vi "D-O Status Module.vi"(8 "error in (no error)":errorcluster, 11 "?":T1={"State"=enum."Idle", "Start Time"=timestamp(0 s since 1904-01-01), "Configuration"={"D-O State"=0, "Cycle Period"=0.0, "DAQmx Task Name"="", "Input Channel Tag Name"=""}, "Current Time"=timestamp(0 s since 1904-01-01), "First Iteration"=FALSE, "Data"={"D-O State"=0}, "Process Name"="", "Pump On?"=enum."Off", "Output Error"=FALSE, "Log Started"=FALSE} {"Data"."D-O State" items=["Default", "On", "Off", "Not Initialized"]; "Configuration"."D-O State" items=["Default", "On", "Off", "Not Initialized"]}) -> (0 "error out":errorcluster, 3 "State out":T1={"State"=enum."Idle", "Start Time"=timestamp(0 s since 1904-01-01), "Configuration"={"D-O State"=0, "Cycle Period"=0.0, "DAQmx Task Name"="", "Input Channel Tag Name"=""}, "Current Time"=timestamp(0 s since 1904-01-01), "First Iteration"=FALSE, "Data"={"D-O State"=0}, "Process Name"="", "Pump On?"=enum."Off", "Output Error"=FALSE, "Log Started"=FALSE} {"Data"."D-O State" items=["Default", "On", "Off", "Not Initialized"]; "Configuration"."D-O State" items=["Default", "On", "Off", "Not Initialized"]})   [LabVIEW 2018, in "D-O Module.lvlib"]
uses:
  D-O Module.lvlib
  Ismatec ISM 831C/Ismatec ISM 831C.lvlib
  Masterflex 7550-30/Masterflex 7550-30.lvlib
  Tag VIs/Tag FGV Operation Enum.ctl
  Shared Variables/Dynamic Shared Variables.lvlib
  Measure Instrument/D-O Module Engine.lvlib
  Tacmina QI/Tacmina QI.lvlib
  KNF Pump/KNF SIMDOS.lvlib
  VICI M50 Party Mode/VICI M50 Party Mode.lvlib
  ASIA Pump.lvlib
  Measure Instrument/State Enum.ctl
  D-O Module Settings Cluster.ctl
  Measure Instrument/State Cluster.ctl
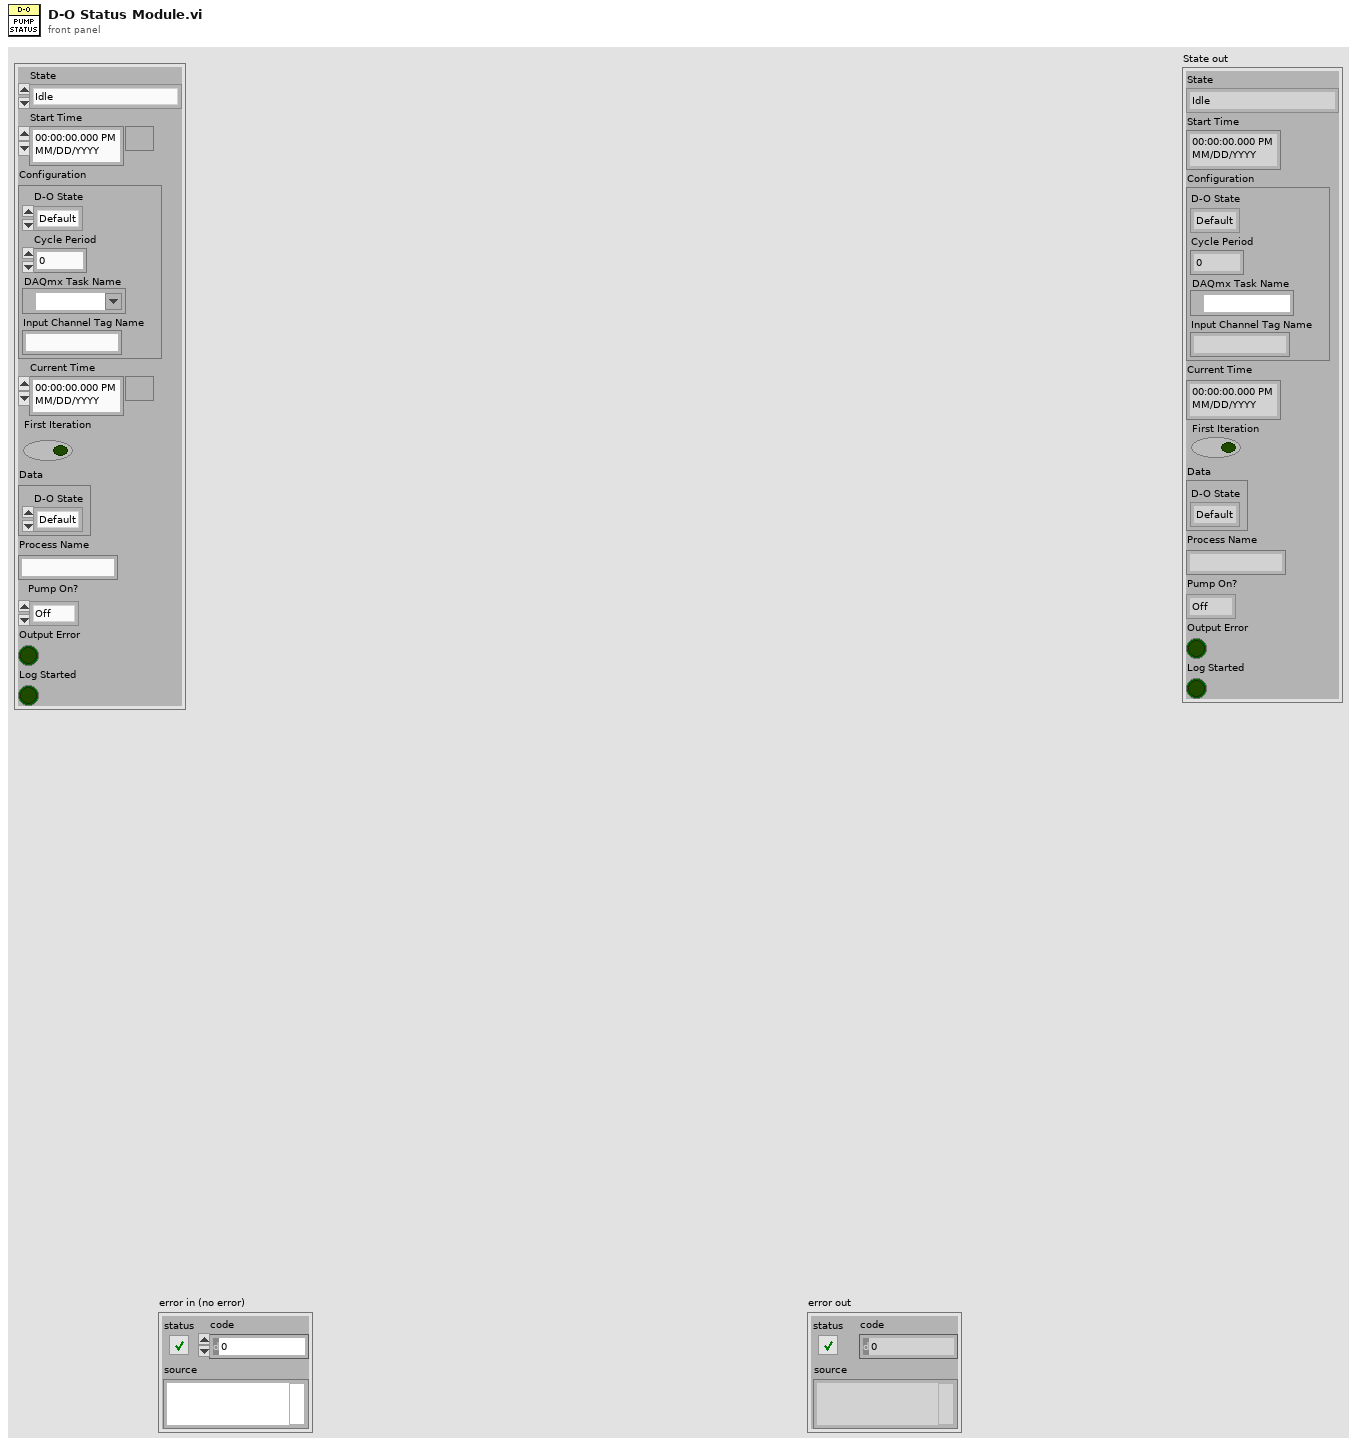
[diagram p1: front panel]
types:
  T1 = typedef "D-O Module.lvlib/D-O Module Engine.lvlib/State Cluster.ctl" = cluster{"State":T2, "Start Time":timestamp, "Configuration":T3, "Current Time":timestamp, "First Iteration":bool, "Data":cluster{"D-O State":u16}, "Process Name":string, "Pump On?":enum16{"Off", "On", "Not Initialized"}, "Output Error":bool, "Log Started":bool}
  T2 = typedef "D-O Module.lvlib/D-O Module Engine.lvlib/State Enum.ctl" = enum16{"Measuring", "Idle", "Paused"}
  T3 = typedef "D-O Module.lvlib/D-O Module Settings Cluster.ctl" = cluster{"D-O State":u16, "Cycle Period":dbl, "DAQmx Task Name":refnum<k21>, "Input Channel Tag Name":string}
  T4 = typedef "Tag FGV Operation Enum.ctl" = enum16{"Init", "Set Notification Queue", "Create Tag", "Commit", "Write Tag (Numeric)", "Write Tag (Boolean)", "Read All Tags", "Read One Tag", "Delete Tag Category", "Set Alarm Parameters (Numeric)", "Set Alarm Parameters (Boolean)", "Enable All Alarms", "Disable All Alarms", "Delete All Tags", "Read Alarms", "Ack Alarm"}
  T5 = typedef "PID 2 Output Enum.ctl" = enum16{"Default", "Ismatec ISM 831C", "Masterflex 7550-30", "VICI M50", "Tacmina QI", "KNF SIMDOS", "ASIA Type C"}
  T6 = typedef "Masterflex 7550-30.lvlib/Settings Cluster.ctl" = cluster{"VISA resource name":refnum<visa-resource-name>, "Simulated?":bool, "Pump Number":dbl, "Reverse?":bool}
  T7 = typedef "Ismatec ISM 831C.lvlib/Ismatech Settings Cluster.ctl" = cluster{"VISA resource name":refnum<visa-resource-name>, "Simulated?":bool, "Pump Number":dbl, "Reverse?":bool}
  T8 = typedef "VICI M50 Party Mode.lvlib/Settings Cluster.ctl" = cluster{"VISA resource name":refnum<visa-resource-name>, "Simulated?":bool, "Pump Letter":string, "Reverse?":bool}
  T9 = typedef "Tacmina QI.lvlib/Tacmina QI DAQ Setting.ctl" = cluster{"Analog DAQ Task":refnum<k21>, "Digital DAQ Task":refnum<k21>}
  T10 = typedef "KNF SIMDOS.lvlib/Settings Cluster plus SIMDOS.ctl" = cluster{"VISA resource name":refnum<visa-resource-name>, "Simulated?":bool}
  T11 = typedef "ASIA Pump.lvlib/Pump Settings.ctl" = cluster{"ASIA Pump #":i32, "channel":i32, "Simulated":bool}
  T12 = typedef "D-O Module.lvlib/D-O Module Tag Names Cluster.ctl" = cluster{"D-O Status":string, "Output Device Tag":string}
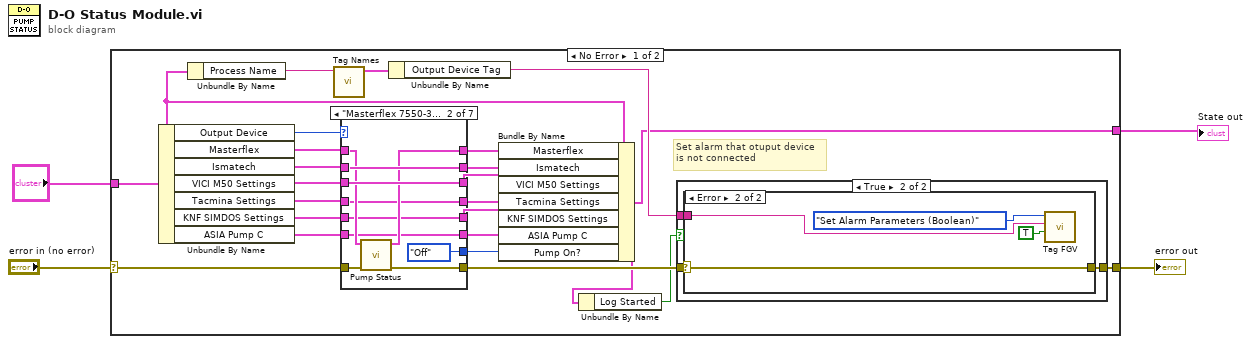
[diagram p0: block diagram]
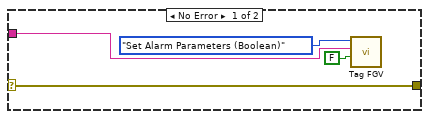
[diagram p3: hidden frame]
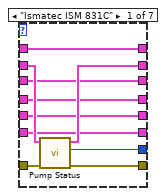
[diagram p4: hidden frame]
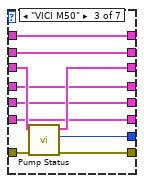
[diagram p5: hidden frame]
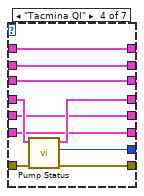
[diagram p6: hidden frame]
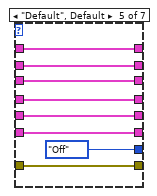
[diagram p7: hidden frame]
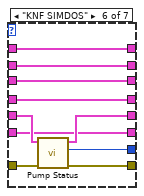
[diagram p8: hidden frame]
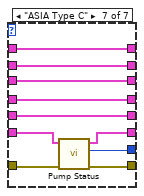
[diagram p9: hidden frame]
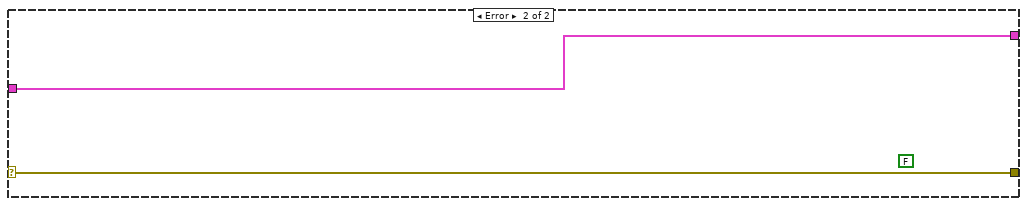
[diagram p10: hidden frame]
diagram:
  n1 = case shown="No Error" "error in (no error)" {
    selector: "error in (no error)" -> [w23 w109]
    tunnel: [w20 w109] -> w3
    tunnel: "?" -> [w19 w108]
    tunnel: [w6 w108] -> w1
    frame No Error {
      # "Set alarm that otuput device\nis not connected"
      n2 = Unbundle By Name(w19) -> ("Output Device"=w15:T5, "Masterflex"=w12:T6, "Ismatech"=w14:T7, "VICI M50 Settings"=w25:T8, "Tacmina Settings"=w16:T9, "KNF SIMDOS Settings"=w10:T10, "ASIA Pump C"=w7:T11)
      n3 = Unbundle By Name(w19) -> ("Process Name"=w17:string)
      n4 = call "Tag Names.vi"("Process Name"=w17) -> ("Pump Module Tag Names"=w18:T12)  [unwired: 8 in, 2 out]
      n5 = case shown="\"Masterflex 7550-30\"" w15 {
        tunnel: w12 -> [w49 w54 w68 w79 w87 w97 w107]
        tunnel: [w49 w55 w68 w79 w87 w97 w107] -> w27
        tunnel: w14 -> [w46 w59 w69 w78 w86 w96 w106]
        tunnel: [w47 w56 w64 w74 w84 w92 w101] -> w21
        tunnel: w23 -> [w48 w57 w65 w75 w84 w93 w102]
        tunnel: [w45 w59 w69 w78 w86 w96 w106] -> w26
        tunnel: w25 -> [w43 w58 w66 w77 w85 w95 w105]
        tunnel: [w43 w58 w67 w77 w85 w95 w105] -> w24
        tunnel: w16 -> [w44 w53 w63 w76 w83 w94 w104]
        tunnel: [w44 w53 w63 w73 w83 w94 w104] -> w13
        tunnel: [w42 w52 w62 w72 w82 w91 w103] -> w11
        tunnel: w10 -> [w42 w52 w62 w72 w82 w90 w103]
        tunnel: [w41 enum16{"Off", "On", "Not Initialized"}."Off" ("Pump On?") w61 w71 enum16{"Off", "On", "Not Initialized"}."Off" ("Pump On?") w89 w100] -> w9
        tunnel: [w40 w50 w60 w70 w80 w88 w99] -> w8
        tunnel: w7 -> [w40 w50 w60 w70 w80 w88 w98]
        frame "Ismatec ISM 831C" {
          n6 = call "Pump Status.vi"("error in (no error)"=w48, "Ismatech Settings"=w46) -> ("error out"=w47:errorcluster, "Pump On?"=w41:enum16{"Off", "On", "Not Initialized"}, "Ismatech Settings"=w45:T7)  [unwired: 6 in, 1 out]
        }
        frame "Masterflex 7550-30" {
          n7 = call "Pump Status.vi"("error in (no error)"=w57, "Masterflex Settings in"=w54) -> ("error out"=w56:errorcluster, "Masterflex Settings out"=w55:T6)  [unwired: 6 in, 2 out]
        }
        frame "VICI M50" {
          n8 = call "Pump Status.vi"("error in (no error)"=w65, "VICI Settings"=w66) -> ("error out"=w64:errorcluster, "Pump On?"=w61:enum16{"Off", "On", "Not Initialized"}, "VICI Settings"=w67:T8)  [unwired: 6 in, 1 out]
        }
        frame "Tacmina QI" {
          n9 = call "Pump Status.vi"("error in"=w75, "Tacmina Settings in"=w76) -> ("error out"=w74:errorcluster, "Pump On?"=w71:enum16{"Off", "On", "Not Initialized"}, "Tacmina Settings out"=w73:T9)  [unwired: 6 in, 1 out]
        }
        frame "Default", Default {
        }
        frame "KNF SIMDOS" {
          n10 = call "Pump Status.vi"("error in (no error)"=w93, "KNF Settings"=w90) -> ("error out"=w92:errorcluster, "Pump On?"=w89:enum16{"Off", "On", "Not Initialized"}, "KNF Settings"=w91:T10)  [unwired: 6 in, 1 out]
        }
        frame "ASIA Type C" {
          n11 = call "Pump Status.vi"("error in (no error)"=w102, "ASIA Pump C Settings in"=w98) -> ("error out"=w101:errorcluster, "Pump On?"=w100:enum16{"Off", "On", "Not Initialized"}, "ASIA Pump C Settings out"=w99:T11)  [unwired: 4 in, 3 out]
        }
      }
      n12 = Unbundle By Name(w18) -> ("Output Device Tag"=w22:string)
      n13 = Bundle By Name(cluster=w19, "Masterflex"=w27, "Ismatech"=w26, "VICI M50 Settings"=w24, "Tacmina Settings"=w13, "KNF SIMDOS Settings"=w11, "ASIA Pump C"=w8, "Pump On?"=w9) -> (w6:T1)
      n14 = Unbundle By Name(w6) -> ("Log Started"=w5:bool)
      n15 = case shown="True" w5 {
        tunnel: w22 -> [_ w31]
        tunnel: w21 -> [w28 w30]
        tunnel: [w28 w29] -> w20
        frame False {
        }
        frame True {
          n16 = case shown="Error" w30 {
            selector: w30 -> [w35 w39]
            tunnel: [w35 w39] -> w29
            tunnel: w31 -> [w32 w38]
            frame No Error {
              n17 = call "Tag FGV.vi"("Data"=FALSE, "Tag Name"=w32, "Operation"=Tag_FGV_Operation_Enum."Set Alarm Parameters (Boolean)") -> ()  [unwired: 3 in, 6 out]
            }
            frame Error {
              n18 = call "Tag FGV.vi"("Data"=TRUE, "Tag Name"=w38, "Operation"=Tag_FGV_Operation_Enum."Set Alarm Parameters (Boolean)") -> ()  [unwired: 3 in, 6 out]
            }
          }
        }
      }
    }
    frame Error {
      (unwired) FALSE
    }
  }
  "error out" <- w3
  "State out" <- w1
